vi "Filter Wheel Simulate New Position.vi"(9 "Velocity (cnts/sec)":dbl, 10 "Position":dbl, 11 "Axis Status":T1) -> (1 "move complete":bool, 2 "New Pos":dbl, 3 "Axis Status Out":T1)   [LabVIEW 2021, in "Filter Wheel Simulator.lvclass"]
uses:
  Filter Wheel Simulator.lvclass
  Filter Wheel cluster Simulated Status.ctl
  Filter Wheel Simulator.lvclass/Filter Wheel Simulator.ctl
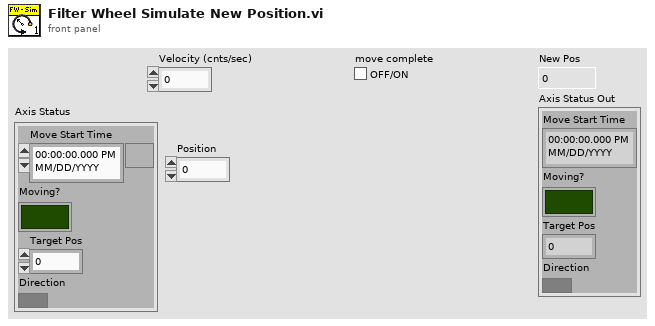
[diagram p1: front panel]
types:
  T1 = typedef "Filter Wheel Simulator.lvclass/Filter Wheel cluster Simulated Status.ctl" = cluster{"Move Start Time":timestamp, "Moving?":bool, "Target Pos":dbl, "Direction":bool}
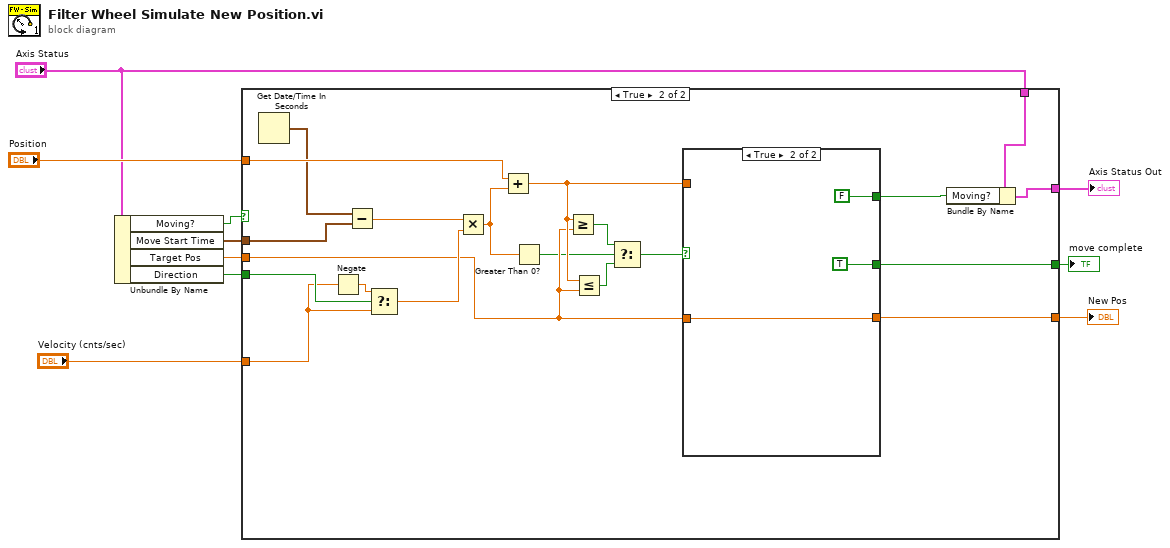
[diagram p0: block diagram]
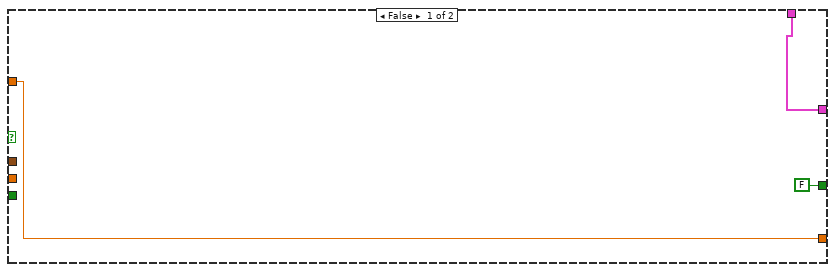
[diagram p2: hidden frame]
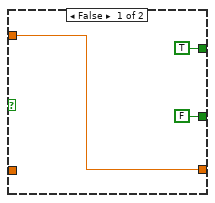
[diagram p3: hidden frame]
diagram:
  n1 = Unbundle By Name("Axis Status") -> ("Moving?"=w2:bool, "Move Start Time"=w10:timestamp, "Target Pos"=w6:dbl, "Direction"=w9:bool)
  n2 = case shown="True" w2 {
    tunnel: w10 -> [_ w33]
    tunnel: w9 -> [_ w31]
    tunnel: "Velocity (cnts/sec)" -> [_ w30]
    tunnel: "Position" -> [w12 w27]
    tunnel: w6 -> [_ w19]
    tunnel: "Axis Status" -> [w13 w26]
    tunnel: [w13 w24] -> w4
    tunnel: [w12 w22] -> w3
    tunnel: [FALSE w14] -> w1
    frame False {
    }
    frame True {
      n3 = Get Date/Time In Seconds() -> (seconds since 1Jan1904=w23:timestamp)
      n4 = Negate(x=w30) -> (-x=w29:dbl)
      n5 = Subtract(x=w23, y=w33) -> (x-y=w32:dbl)
      n6 = Select(t=w29, s=w31, f=w30) -> (s? t:f=w28:dbl)
      n7 = Multiply(x=w32, y=w28) -> (x*y=w21:dbl)
      n8 = Add(x=w27, y=w21) -> (x+y=w20:dbl)
      n9 = Greater Than 0?(x=w21) -> (x > 0?=w17:bool)
      n10 = Greater Or Equal?(x=w20, y=w19) -> (x >= y?=w16:bool)
      n11 = Less Or Equal?(x=w20, y=w19) -> (x <= y?=w18:bool)
      n12 = Select(t=w16, s=w17, f=w18) -> (s? t:f=w15:bool)
      n13 = case shown="True" w15 {
        tunnel: w20 -> [w36 _]
        tunnel: w19 -> [_ w38]
        tunnel: [TRUE FALSE] -> w25
        tunnel: [w36 w38] -> w22
        tunnel: [FALSE TRUE] -> w14
        frame False {
        }
        frame True {
        }
      }
      n14 = Bundle By Name(cluster=w26, "Moving?"=w25) -> (w24:T1)
    }
  }
  "Axis Status Out" <- w4
  "New Pos" <- w3
  "move complete" <- w1
